vi "Count Shots.vi"(10 "Boolean in":bool, 11 "Value":bool) -> (3 "Boolean out":bool)   [LabVIEW 2012]
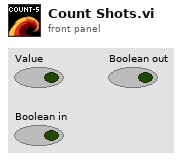
[diagram p1: front panel]
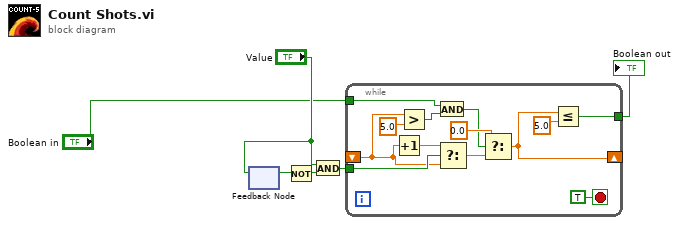
[diagram p0: block diagram]
diagram:
  n1 = feedback #1() -> (w5:bool)  [unwired: 1 in]
  n2 = feedback-in #1("Value") -> ()
  n3 = Not(x=w5) -> (.not. x?=w4:bool)
  n4 = And(x="Value", y=w4) -> (x .and. y?=w3:bool)
  n5 = while {
    tunnel: w3 -> [w15]
    tunnel: "Boolean in" -> [w11]
    shift-right: [w9] -> _
    shift-left: _ -> [w14]
    tunnel: [w7] -> w2
    stop <- TRUE stop-if-true
    n6 = Increment(x=w14) -> (x+1=w18:dbl)
    n7 = Greater?(x=w14, y=5.0) -> (0:w12:bool)
    n8 = And(x=w11, y=w12) -> (x .and. y?=w10:bool)
    n9 = Select(t=w18, s=w15, f=w14) -> (s? t:f=w17:dbl)
    n10 = Select(t=0.0, s=w10, f=w17) -> (s? t:f=w9:dbl)
    n11 = Less Or Equal?(x=w9, y=5.0) -> (x <= y?=w7:bool)
  }
  "Boolean out" <- w2
